vi "LVCAM Propagate Error.vi"(10 "error in":errorcluster, 11 "Process in":refnum<class "ABD.lvclass">) -> (0 "error out":errorcluster)   [LabVIEW 2021, in "ABD.lvlib" / "ABD.lvclass"]
uses:
  ABD.lvclass
  ABD.lvclass/ABD.ctl
  LVCAM/LVCAM/LVCAM/LVCAM.lvclass
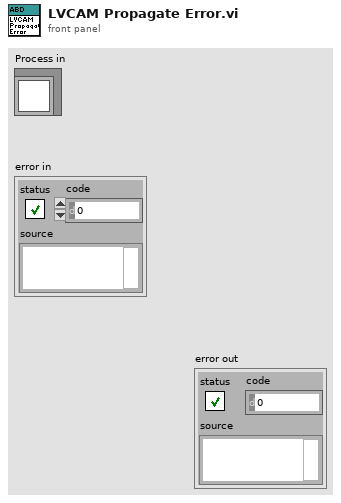
[diagram p1: front panel]
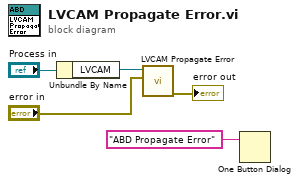
[diagram p0: block diagram]
diagram:
  n1 = Unbundle By Name("Process in") -> ("LVCAM"=w2:refnum<class "LVCAM.lvclass">)
  n2 = call-dynamic "LVCAM Propagate Error.vi"("error in"="error in", "LVCAM Propagate Error in"=w2) -> ("error out"=→"error out":errorcluster)  [unwired: 9 in]
  n3 = One Button Dialog(message="ABD Propagate Error") -> ()  [unwired: 1 in, 1 out]
